vi "Power FGV.vi"(7 "prevent sleep":bool, 8 "error in (no error)":errorcluster, 11 "keep screen on":bool=TRUE) -> (0 "error out":errorcluster)   [LabVIEW 2024, in "Request Power.lvlib"]
uses:
  Request Power.lvlib
  typedefs/Power Request Type.ctl
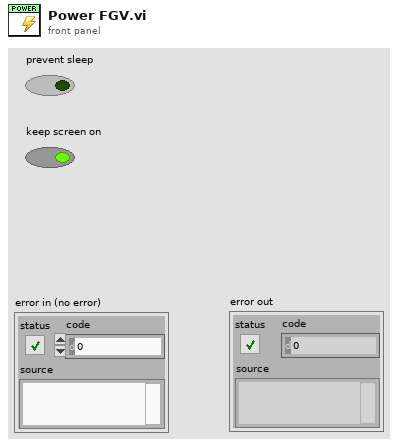
[diagram p1: front panel]
types:
  T1 = typedef "Request Power.lvlib/Power Request Type.ctl" = enum32{"Power Request Display Required", "Power Request System Required", "Power Request Away Mode Required", "Power Request Execution Required"}
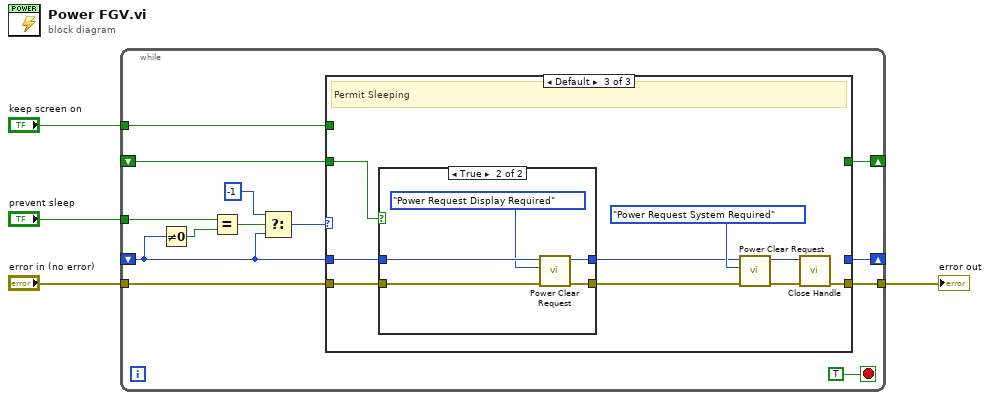
[diagram p0: block diagram]
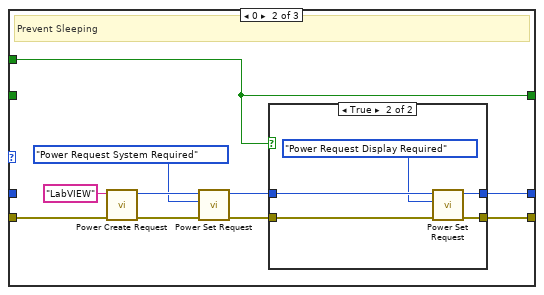
[diagram p3: hidden frame]
diagram:
  n1 = while {
    tunnel: "error in (no error)" -> [w16]
    tunnel: [w15] -> w3
    tunnel: "keep screen on" -> [w14]
    shift-right: [w13] -> _
    shift-left: _ -> [w5]
    shift-right: [w12] -> _
    shift-left: _ -> [w11]
    tunnel: "prevent sleep" -> [w10]
    stop <- TRUE stop-if-true
    n2 = Not Equal To 0?(x=w5) -> (x != 0?=w6:bool)
    n3 = Equal?(x=w10, y=w6) -> (x = y?=w9:bool)
    n4 = Select(t=i64 -1, s=w9, f=w5) -> (s? t:f=w8:i64)
    n5 = case shown="Default" w8 {
      tunnel: w16 -> [w20 w30 w43]
      tunnel: [w20 w23 w44] -> w15
      tunnel: w14 -> [_ w21 _]
      tunnel: [w18 w22 _] -> w13
      tunnel: [w19 w21 _] -> w12
      tunnel: w11 -> [w19 _ w45]
      tunnel: w5 -> [w18 _ w38]
      frame -1 {
        # "Do nothing"
      }
      frame 0 {
        # "Prevent Sleeping"
        n6 = call "Power Create Request.vi"("error in (no error)"=w30, "Simple Reason String"="LabVIEW") -> ("error out"=w28:errorcluster, "Handle"=w27:i64)  [unwired: 7 in, 1 out]
        n7 = call "Power Set Request.vi"("error in (no error)"=w28, "Power Request Type"=Power_Request_Type."Power Request System Required", "Handle in"=w27) -> ("error out"=w25:errorcluster, "Handle out"=w24:i64)  [unwired: 6 in, 1 out]
        n8 = case shown="True" w21 {
          tunnel: w25 -> [w32 w37]
          tunnel: w24 -> [w31 w35]
          tunnel: [w32 w36] -> w23
          tunnel: [w31 w34] -> w22
          frame False {
          }
          frame True {
            n9 = call "Power Set Request.vi"("error in (no error)"=w37, "Power Request Type"=Power_Request_Type."Power Request Display Required", "Handle in"=w35) -> ("error out"=w36:errorcluster, "Handle out"=w34:i64)  [unwired: 6 in, 1 out]
          }
        }
      }
      frame Default {
        # "Permit Sleeping"
        n10 = case shown="True" w45 {
          tunnel: w43 -> [w47 w53]
          tunnel: w38 -> [w48 w52]
          tunnel: [w47 w51] -> w41
          tunnel: [w48 w50] -> w42
          frame False {
          }
          frame True {
            n11 = call "Power Clear Request.vi"("error in (no error)"=w53, "Power Request Type"=Power_Request_Type."Power Request Display Required", "Handle in"=w52) -> ("error out"=w51:errorcluster, "Handle out"=w50:i64)  [unwired: 6 in, 1 out]
          }
        }
        n12 = call "Power Clear Request.vi"("error in (no error)"=w41, "Power Request Type"=Power_Request_Type."Power Request System Required", "Handle in"=w42) -> ("error out"=w39:errorcluster, "Handle out"=w40:i64)  [unwired: 6 in, 1 out]
        n13 = call "Close Handle.vi"("error in (no error)"=w39, "Handle"=w40) -> ("error out"=w44:errorcluster)  [unwired: 8 in, 1 out]
      }
    }
  }
  "error out" <- w3
